vi "getSlotString.vi"(1 "Slot":i32=10 min=0 max=14) -> (0 "string":string)   [LabVIEW 2011]
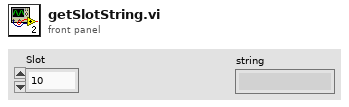
[diagram p1: front panel]
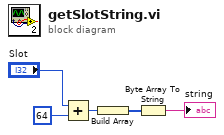
[diagram p0: block diagram]
diagram:
  n1 = Add(x="Slot", y=u32 64) -> (x+y=w5:u32)
  n2 = Build Array(w5) -> (w4:u32[])
  n3 = Byte Array To String(unsigned byte array=w4) -> (string=→"string":string)
